vi "Get Boolean Variable.vi"(8 "error in (no error)":errorcluster, 10 "Name":string, 11 "Application in":refnum<class "Application.lvclass">) -> (0 "error out":errorcluster, 2 "Value":bool, 3 "Application out":refnum<class "Application.lvclass">)   [LabVIEW 2017, in "Application.lvlib" / "Application.lvclass"]
doc: "Retrieves a named variable from the local variable engine and casts it as a boolean."
uses:
  Application.lvclass
  <vilib>/TSS/ACRObat Test Framework/Classes/Variable Engine/Class/Variable Engine.lvclass
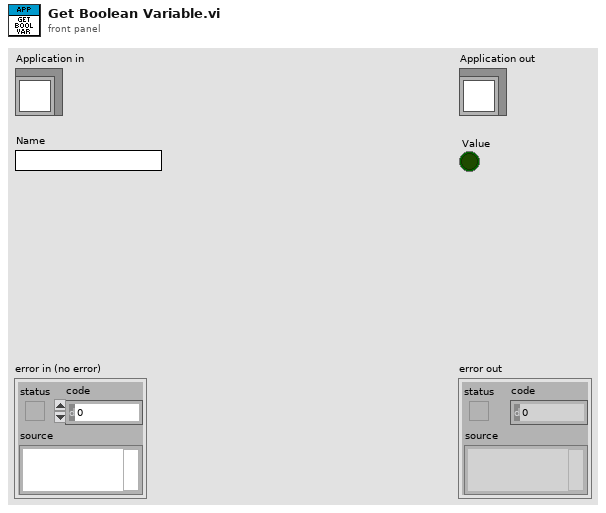
[diagram p1: front panel]
types:
  T1 = typedef "Application.lvlib/App Properties.lvclass/Class Properties -- Cluster.ctl" = cluster{"UUT Info":T2[], "Test Information":refnum<vi>, "Gold Board":refnum<class "Golden Board.lvclass">, "Test Recipe":refnum<class "Test Recipe.lvclass">, "Instruments":refnum<class "Instrument.lvclass">[], "Mode":T3, "Test Results":T4[], "Station Config":refnum<class "Station Config.lvclass">, "Variable Engine":refnum<class "Variable Engine.lvclass">}
  T2 = typedef "Application.lvlib/App Properties.lvclass/UUT Reference -- Cluster.ctl" = cluster{"Serial Number Reference":refnum<vi>, "Status Message Reference":refnum<vi>}
  T3 = typedef "Application.lvlib/Application.lvclass/Op Mode -- Enum.ctl" = u16
  T4 = typedef "Application.lvlib/App Properties.lvclass/Test Result -- Cluster.ctl" = cluster{"Position":i32, "Pass":bool, "Fail Codes":string}
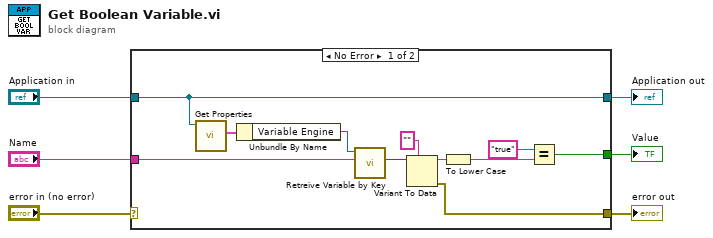
[diagram p0: block diagram]
diagram:
  n1 = case shown="No Error" "error in (no error)" {
    selector: "error in (no error)" -> [_ w19]
    tunnel: [w11 w19] -> w5
    tunnel: [w14 w18] -> w3
    tunnel: "Application in" -> [w14 w18]
    tunnel: "Name" -> [w16 _]
    tunnel: [w7 _] -> w1
    frame No Error {
      n2 = call "Get Properties.vi"("Acrobat Template in"=w14) -> ("Class Properties"=w13:T1)  [unwired: 8 in, 2 out]
      n3 = Unbundle By Name(w13) -> ("Variable Engine"=w12:refnum<class "Variable Engine.lvclass">)
      n4 = call <vilib>:"Retreive Variable by Key.vi"("Key"=w16, "Acrobat Template in"=w12) -> ("Value"=w17:variant)  [unwired: 7 in, 2 out]
      n5 = Variant To Data(type="" ("Value"), Variant=w17) -> (data=w15:string, error out=w11:errorcluster)  [unwired: 1 in]
      n6 = To Lower Case(string=w15) -> (all lower case string=w8:string)
      n7 = Equal?(x="true", y=w8) -> (x = y?=w7:bool)
    }
    frame Error {
    }
  }
  "error out" <- w5
  "Application out" <- w3
  "Value" <- w1
